vi "SetTriggerTimer.vi"(8 "Error In":errorcluster, 10 "Interval (sec)":dbl, 11 "Keithley 7001 In":refnum<visa-resource-name>) -> (0 "Error Out":errorcluster, 3 "Keithley 7001 Out":refnum<visa-resource-name>)   [LabVIEW 2012, in "Keithley-7001.lvlib"]
uses:
  Keithley-7001.lvlib
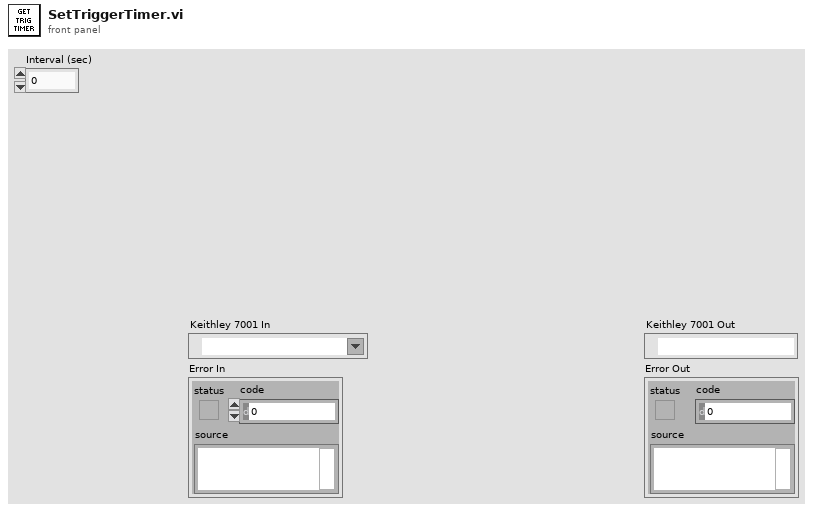
[diagram p1: front panel]
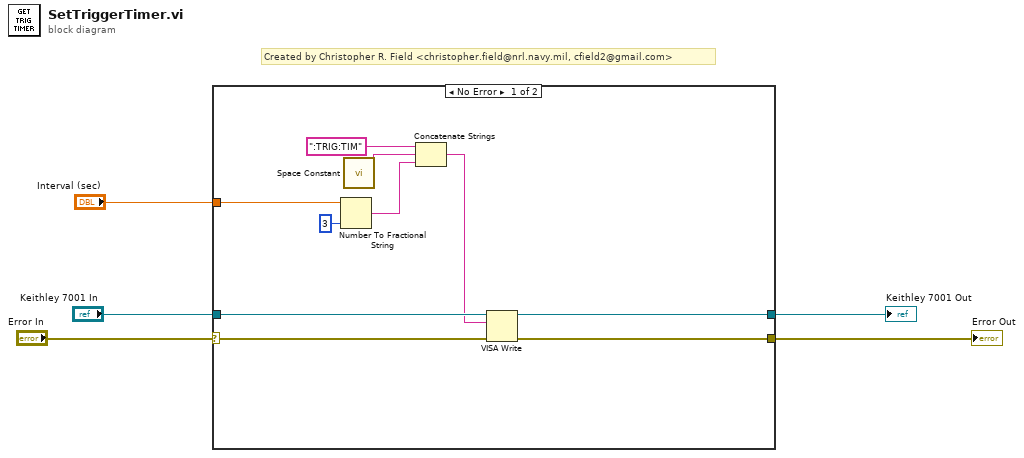
[diagram p0: block diagram]
diagram:
  # "Created by Christopher R. Field <christopher.field@nrl.navy.mil, cfield2@gmail.com>"
  n1 = case shown="No Error" "Error In" {
    selector: "Error In" -> [w6 w16]
    tunnel: "Keithley 7001 In" -> [w15 w17]
    tunnel: [w14 w17] -> w4
    tunnel: [w13 w16] -> w3
    tunnel: "Interval (sec)" -> [w9 _]
    frame No Error {
      n2 = Number To Fractional String(number=w9, precision (6)=i16 3) -> (F-format string=w8:string)  [unwired: 2 in]
      n3 = call <vilib>:"Space Constant.vi"() -> ("String"=w11:string)
      n4 = Concatenate Strings(":TRIG:TIM" ("write buffer"), w11, w8) -> (w10:string)
      n5 = VISA Write(VISA resource name=w15, write buffer=w10, error in (no error)=w6) -> (VISA resource name out=w14:refnum<visa-resource-name>, error out=w13:errorcluster)  [unwired: 1 out]
    }
    frame Error {
    }
  }
  "Keithley 7001 Out" <- w4
  "Error Out" <- w3
